vi "power_supply_FSM.vi"(0 "measurements q":refnum<queue>, 1 "commands q":refnum<queue>, 2 "GPIB":string, 3 "MAX_CURR":dbl, 4 "OUT_CURR":dbl, 5 "STEP":dbl=0.1, 7 "error in (no error)":errorcluster) -> ()   [LabVIEW 2019]
panel:
  out "state_and_args":string
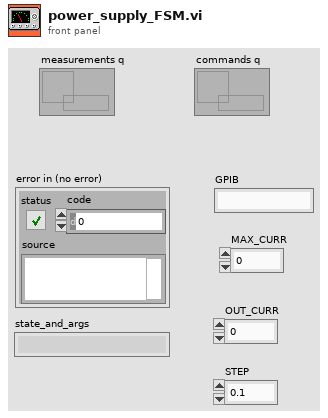
[diagram p1: front panel]
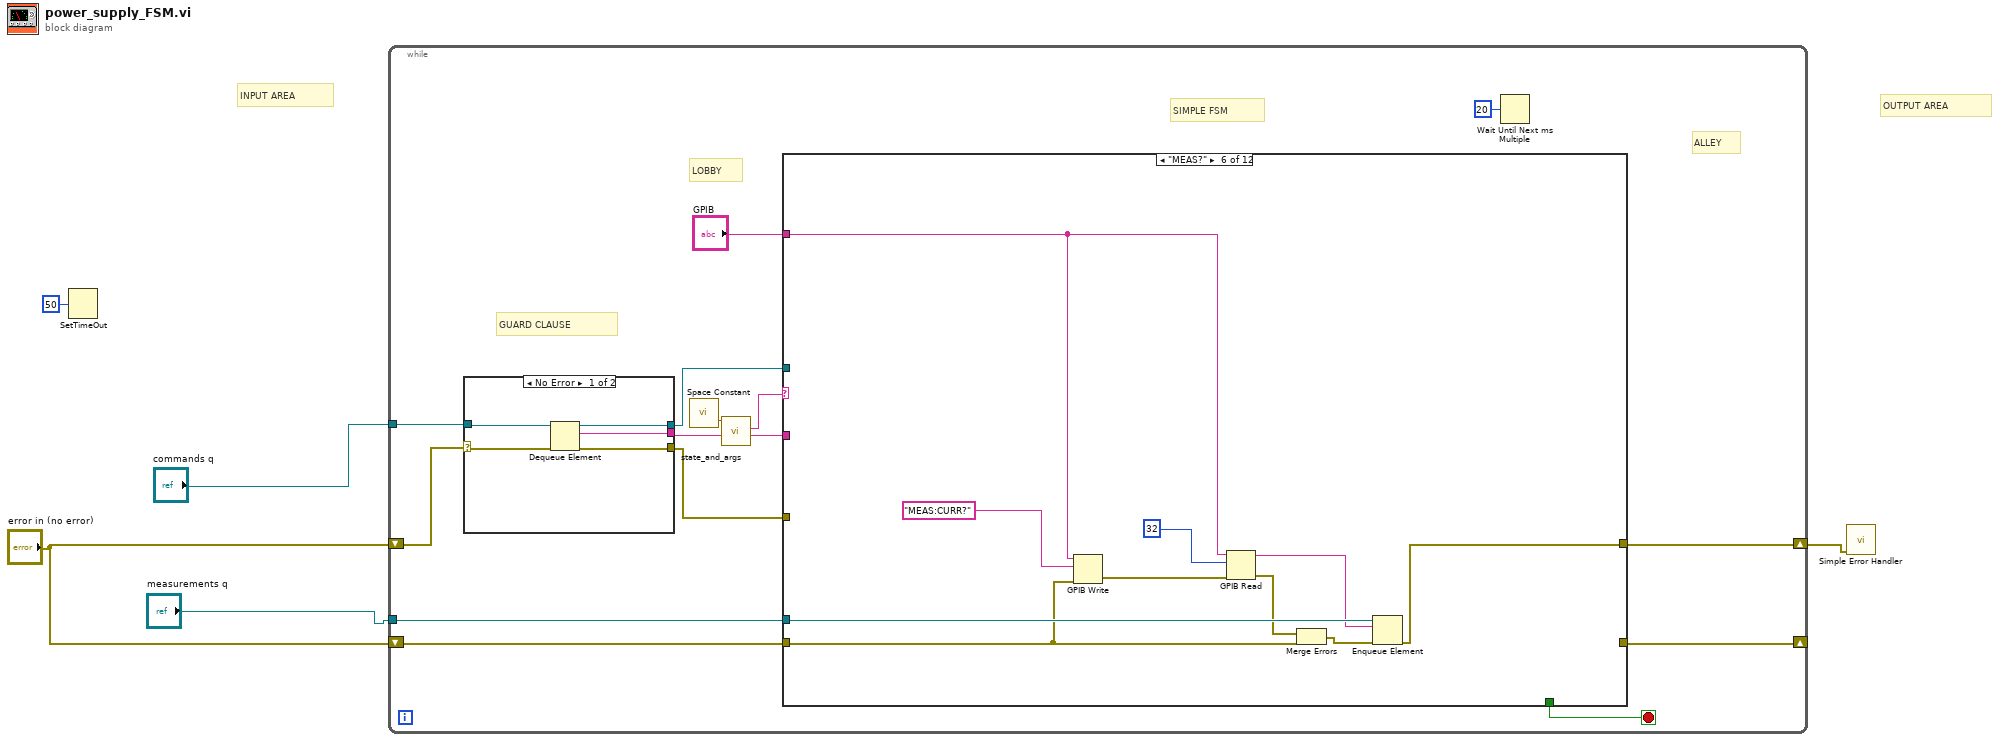
[diagram p0: block diagram]
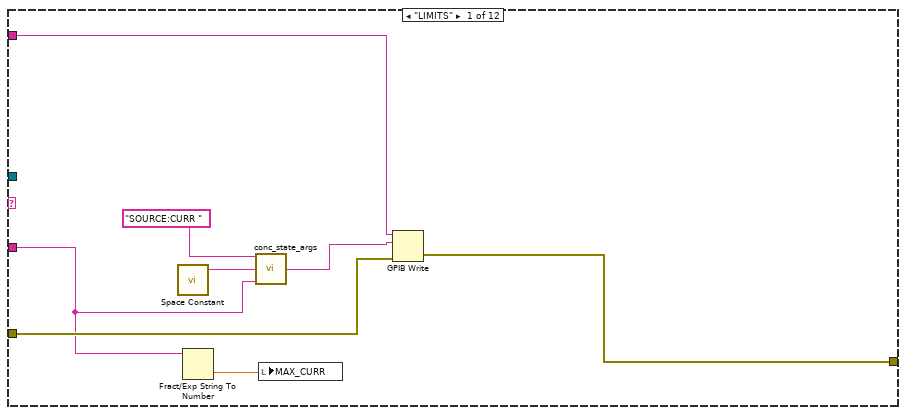
[diagram p2: hidden frame]
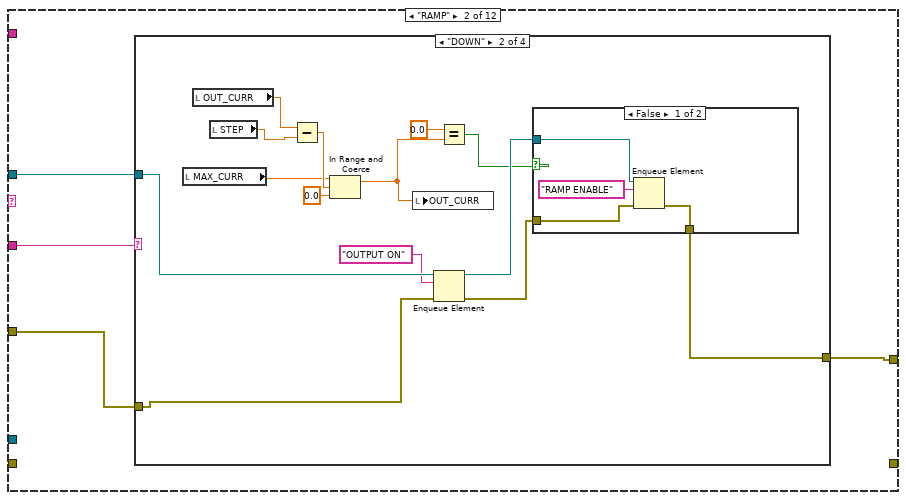
[diagram p3: hidden frame]
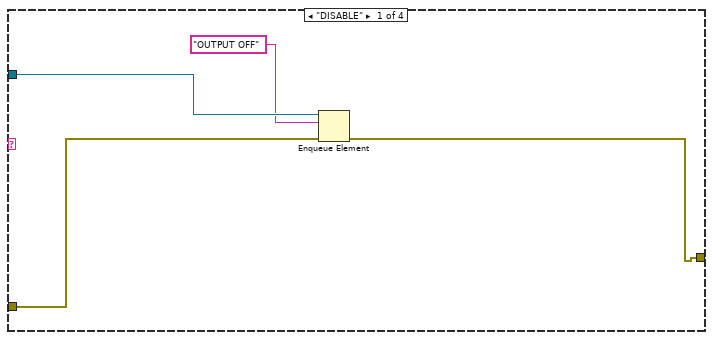
[diagram p4: hidden frame]
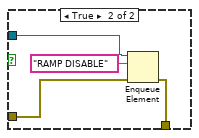
[diagram p5: hidden frame]
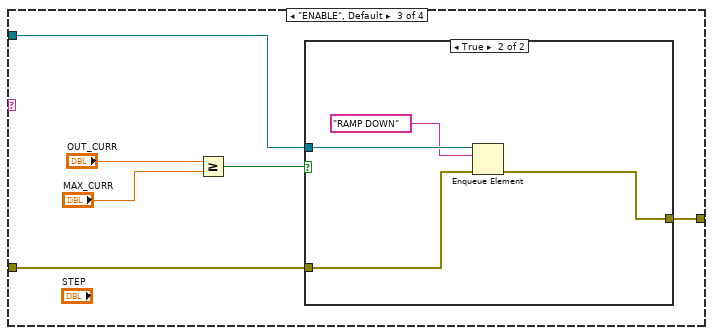
[diagram p6: hidden frame]
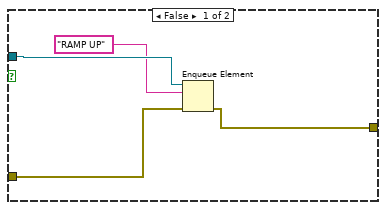
[diagram p7: hidden frame]
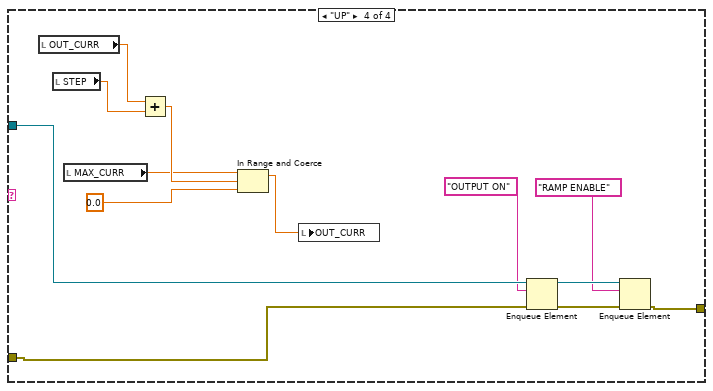
[diagram p8: hidden frame]
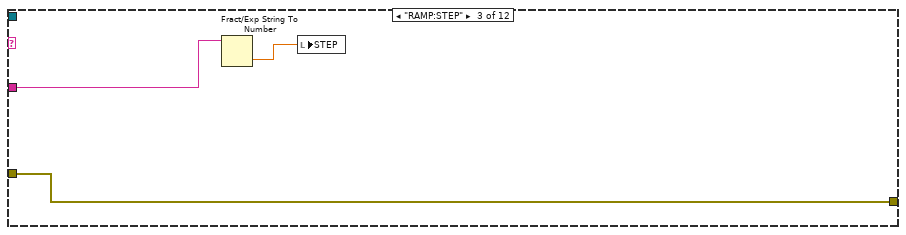
[diagram p9: hidden frame]
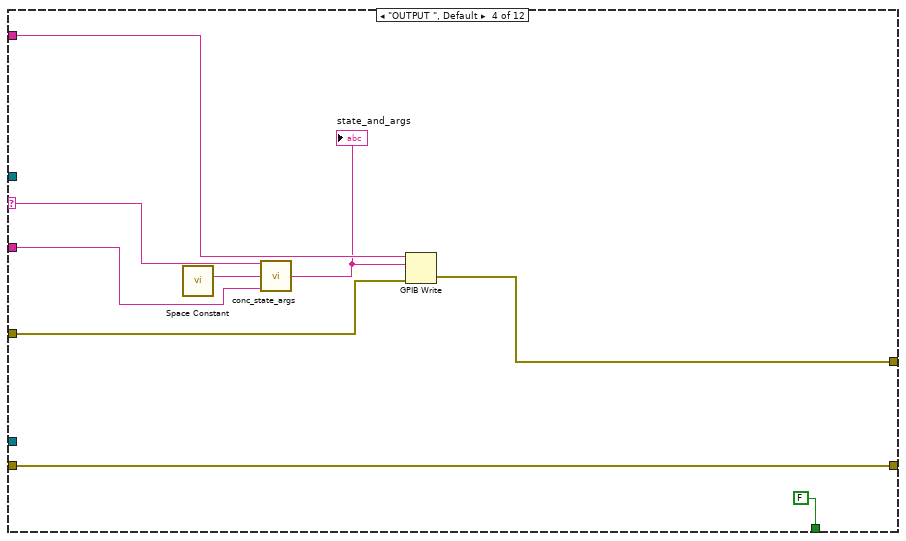
[diagram p10: hidden frame]
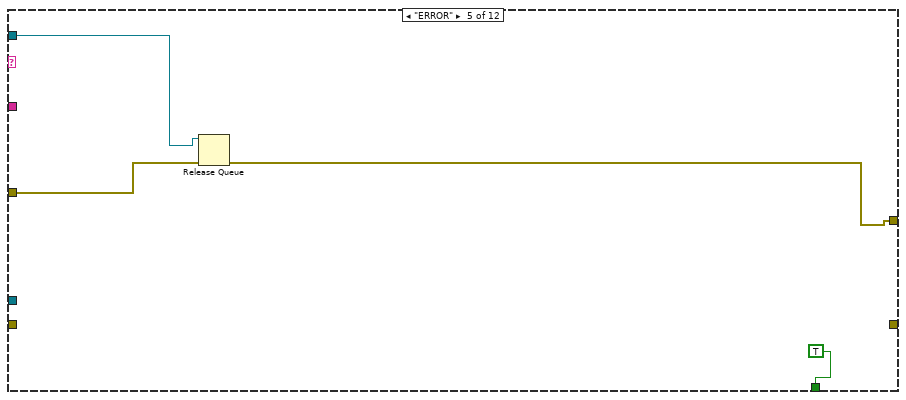
[diagram p11: hidden frame]
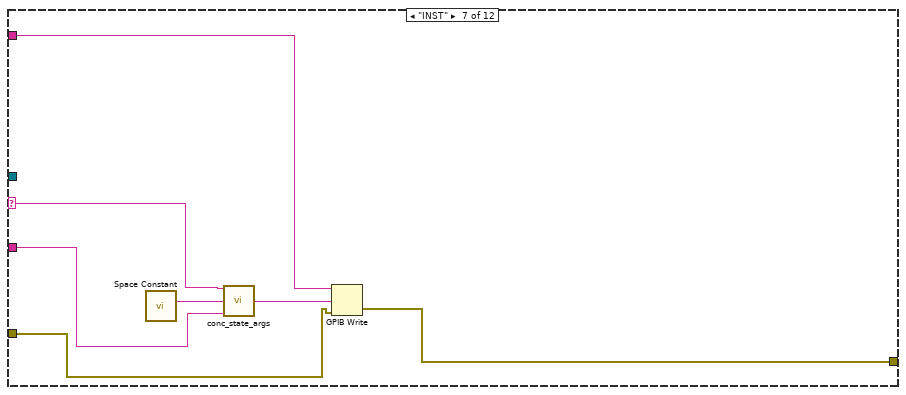
[diagram p12: hidden frame]
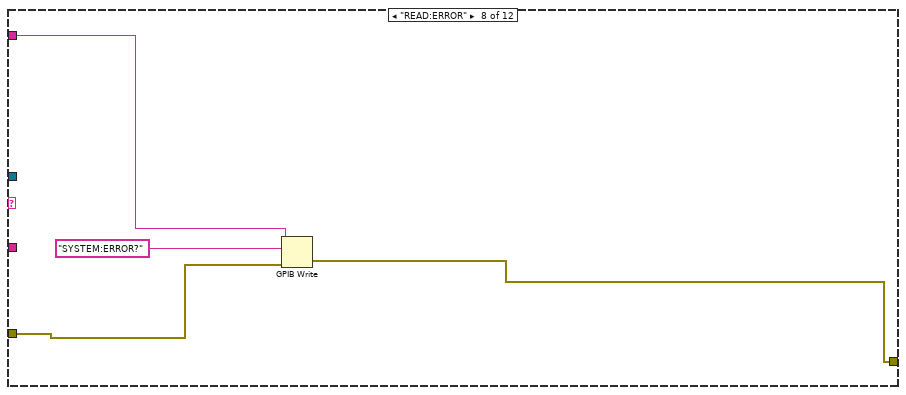
[diagram p13: hidden frame]
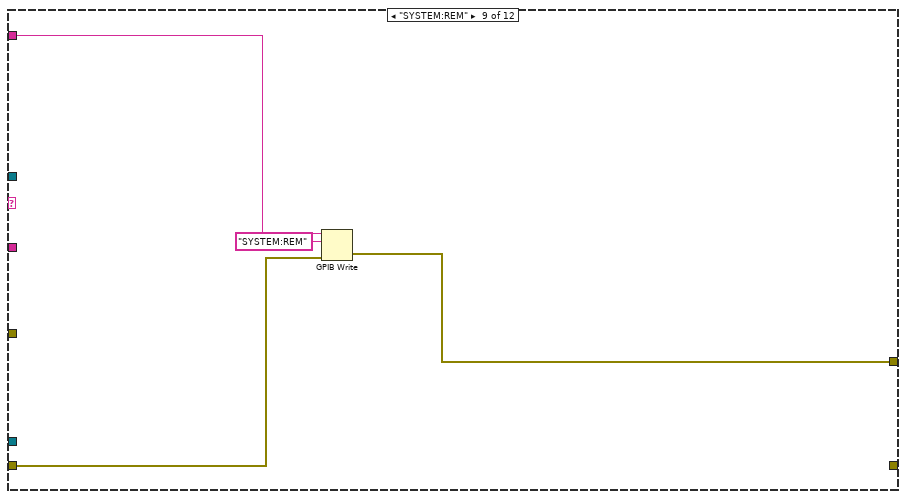
[diagram p14: hidden frame]
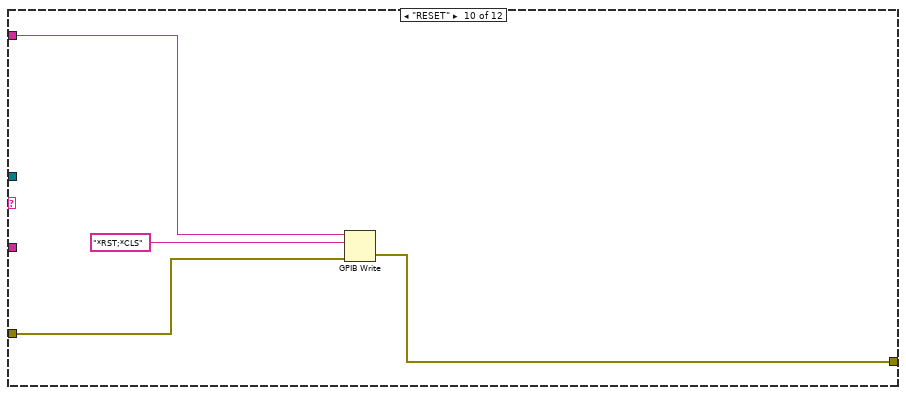
[diagram p15: hidden frame]
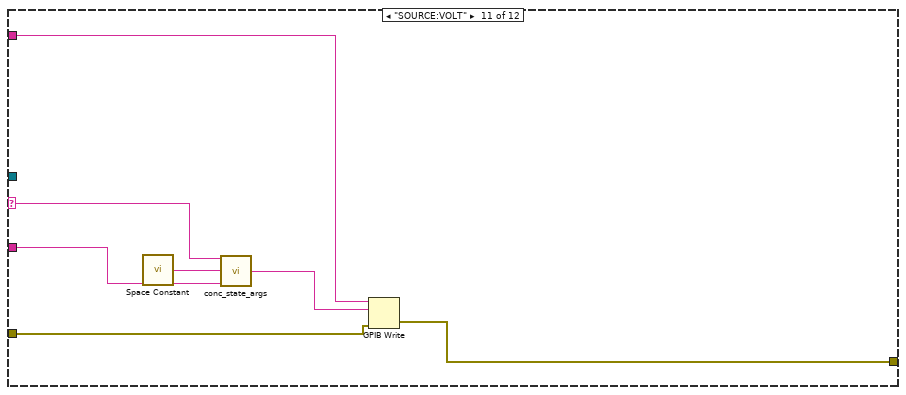
[diagram p16: hidden frame]
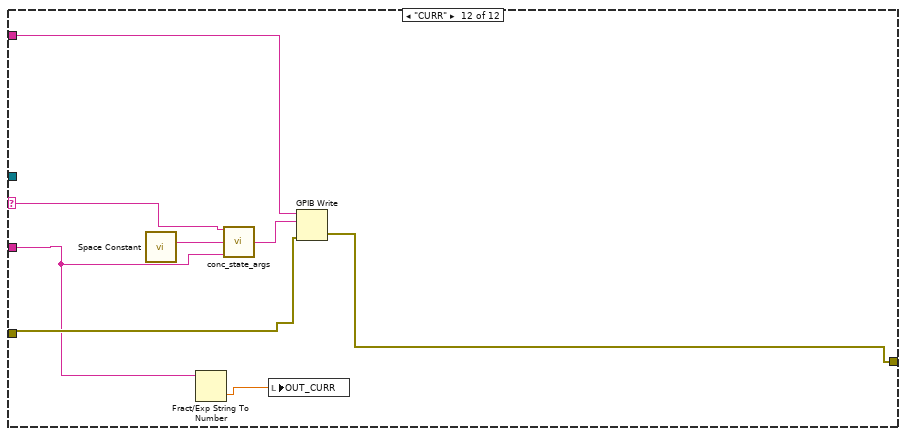
[diagram p17: hidden frame]
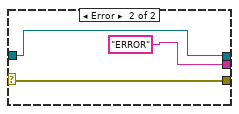
[diagram p18: hidden frame]
diagram:
  # "OUTPUT AREA"
  # "INPUT AREA"
  n1 = SetTimeOut(1:50 ("new timeout (10000)")) -> ()  [unwired: 1 out]
  n2 = while {
    tunnel: "commands q" -> [w19]
    shift-right: [w12] -> w4
    shift-left: "error in (no error)" -> [w20]
    shift-right: [w7] -> _
    shift-left: "error in (no error)" -> [w9]
    tunnel: "measurements q" -> [w8]
    stop <- w10 stop-if-true
    # "SIMPLE FSM"
    # "ALLEY"
    # "LOBBY"
    # "GUARD CLAUSE"
    n3 = case shown="No Error" w20 {
      selector: w20 -> [w149 w151]
      tunnel: w19 -> [w150 w152]
      tunnel: [w148 w152] -> w11
      tunnel: [w147 w151] -> w15
      tunnel: [w146 "ERROR"] -> w18
      frame No Error {
        n4 = Dequeue Element(queue=w150, error in (no error)=w149) -> (queue out=w148:refnum<queue>, element=w146:string, error out=w147:errorcluster)  [unwired: 1 in, 1 out]
      }
      frame Error {
      }
    }
    n5 = call <vilib>:"Space Constant.vi"() -> ("String"=w17:string)
    n6 = call "state_and_args.vi"("String"=w18, "DELIMITER (:)"=w17) -> ("Arguments"=w14:string, "State"=w16:string)  [unwired: 8 in]
    n7 = case shown="\"MEAS?\"" w16 {
      selector: w16 -> [_ _ _ w95 _ _ w115 _ _ _ w136 w143]
      tunnel: w15 -> [w25 w30 w86 w94 w100 _ w114 w120 _ w128 w132 w142]
      tunnel: w14 -> [w22 w32 w88 w97 _ _ w116 _ _ _ w137 w139]
      tunnel: "GPIB" -> [w26 _ _ w96 _ w110 w118 w122 w126 w130 w134 w145]
      tunnel: [w24 w29 w86 w93 w99 w106 w113 w119 w123 w127 w131 w141] -> w12
      tunnel: w11 -> [_ w31 _ _ w101 _ _ _ _ _ _ _]
      tunnel: [_ _ _ FALSE TRUE _ _ _ _ _ _ _] -> w10
      tunnel: w9 -> [_ _ _ w90 _ w105 _ _ w124 _ _ _]
      tunnel: w8 -> [_ _ _ _ _ w107 _ _ _ _ _ _]
      tunnel: [_ _ _ w90 _ _ _ _ _ _ _ _] -> w7
      frame "LIMITS" {
        n8 = call <vilib>:"Space Constant.vi"() -> ("String"=w28:string)
        n9 = Fract/Exp String To Number(string=w22) -> (number=w23:dbl)  [unwired: 3 in, 1 out]
        n10 = call "conc_state_args.vi"("State"="SOURCE:CURR ", "DELIMITER (:)"=w28, "Args"=w22) -> ("state_and_args"=w21:string)  [unwired: 12 in]
        n11 = local write "MAX_CURR"(w23) -> ()
        n12 = GPIB Write(0:w26, 1:w21, 3:w25) -> (6:w24:errorcluster)  [unwired: 2 in, 1 out]
      }
      frame "RAMP" {
        n13 = case shown="\"DOWN\"" w32 {
          tunnel: w31 -> [w36 w45 w60 w83]
          tunnel: w30 -> [w35 w44 w61 w82]
          tunnel: [w33 w37 w59 w77] -> w29
          frame "DISABLE" {
            n14 = Enqueue Element(queue=w36, element="OUTPUT OFF", error in (no error)=w35) -> (error out=w33:errorcluster)  [unwired: 1 in, 2 out]
          }
          frame "DOWN" {
            n15 = local read "MAX_CURR"() -> (w47:dbl)
            n16 = local read "OUT_CURR"() -> (w50:dbl)
            n17 = local read "STEP"() -> (w49:dbl)
            n18 = Subtract(x=w50, y=w49) -> (x-y=w48:dbl)
            n19 = In Range and Coerce(upper limit=w47, x=w48, lower limit=0.0) -> (coerced(x)=w42:dbl)  [unwired: 1 out]
            n20 = local write "OUT_CURR"(w42) -> ()
            n21 = Enqueue Element(queue=w45, element="OUTPUT ON", error in (no error)=w44) -> (queue out=w40:refnum<queue>, error out=w39:errorcluster)  [unwired: 1 in, 1 out]
            n22 = Equal?(x=0.0, y=w42) -> (x = y?=w38:bool)
            n23 = case shown="False" w38 {
              tunnel: w40 -> [w52 w58]
              tunnel: w39 -> [w53 w57]
              tunnel: [w54 w55] -> w37
              frame False {
                n24 = Enqueue Element(queue=w52, element="RAMP ENABLE", error in (no error)=w53) -> (error out=w54:errorcluster)  [unwired: 1 in, 2 out]
              }
              frame True {
                n25 = Enqueue Element(queue=w58, element="RAMP DISABLE", error in (no error)=w57) -> (error out=w55:errorcluster)  [unwired: 1 in, 2 out]
              }
            }
          }
          frame "ENABLE", Default {
            n26 = Greater Or Equal?(x="OUT_CURR", y="MAX_CURR") -> (x >= y?=w62:bool)
            n27 = case shown="True" w62 {
              tunnel: w61 -> [w67 w72]
              tunnel: w60 -> [w68 w71]
              tunnel: [w65 w69] -> w59
              frame False {
                n28 = Enqueue Element(queue=w68, element="RAMP UP", error in (no error)=w67) -> (error out=w65:errorcluster)  [unwired: 1 in, 2 out]
              }
              frame True {
                n29 = Enqueue Element(queue=w71, element="RAMP DOWN", error in (no error)=w72) -> (error out=w69:errorcluster)  [unwired: 1 in, 2 out]
              }
            }
          }
          frame "UP" {
            n30 = local read "OUT_CURR"() -> (w84:dbl)
            n31 = local read "STEP"() -> (w85:dbl)
            n32 = local read "MAX_CURR"() -> (w75:dbl)
            n33 = Add(x=w84, y=w85) -> (x+y=w76:dbl)
            n34 = In Range and Coerce(upper limit=w75, x=w76, lower limit=0.0) -> (coerced(x)=w73:dbl)  [unwired: 1 out]
            n35 = local write "OUT_CURR"(w73) -> ()
            n36 = Enqueue Element(queue=w83, element="OUTPUT ON", error in (no error)=w82) -> (queue out=w80:refnum<queue>, error out=w79:errorcluster)  [unwired: 1 in, 1 out]
            n37 = Enqueue Element(queue=w80, element="RAMP ENABLE", error in (no error)=w79) -> (error out=w77:errorcluster)  [unwired: 1 in, 2 out]
          }
        }
      }
      frame "RAMP:STEP" {
        n38 = Fract/Exp String To Number(string=w88) -> (number=w87:dbl)  [unwired: 3 in, 1 out]
        n39 = local write "STEP"(w87) -> ()
      }
      frame "OUTPUT ", Default {
        n40 = call <vilib>:"Space Constant.vi"() -> ("String"=w92:string)
        n41 = call "conc_state_args.vi"("State"=w95, "DELIMITER (:)"=w92, "Args"=w97) -> ("state_and_args"=w89:string)  [unwired: 12 in]
        "state_and_args" <- w89
        n42 = GPIB Write(0:w96, 1:w89, 3:w94) -> (6:w93:errorcluster)  [unwired: 2 in, 1 out]
      }
      frame "ERROR" {
        n43 = Release Queue(queue=w101, error in (no error)=w100) -> (error out=w99:errorcluster)  [unwired: 1 in, 2 out]
      }
      frame "MEAS?" {
        n44 = GPIB Write(0:w110, 1:"MEAS:CURR?", 3:w105) -> (6:w111:errorcluster)  [unwired: 2 in, 1 out]
        n45 = GPIB Read(0:w110, 1:32 ("byte count"), 3:w111) -> (5:w102:string, 7:w103:errorcluster)  [unwired: 2 in, 1 out]
        n46 = Merge Errors(w103, w105) -> (w108:errorcluster)
        n47 = Enqueue Element(queue=w107, element=w102, error in (no error)=w108) -> (error out=w106:errorcluster)  [unwired: 1 in, 2 out]
      }
      frame "INST" {
        n48 = call <vilib>:"Space Constant.vi"() -> ("String"=w117:string)
        n49 = call "conc_state_args.vi"("State"=w115, "DELIMITER (:)"=w117, "Args"=w116) -> ("state_and_args"=w112:string)  [unwired: 12 in]
        n50 = GPIB Write(0:w118, 1:w112, 3:w114) -> (6:w113:errorcluster)  [unwired: 2 in, 1 out]
      }
      frame "READ:ERROR" {
        n51 = GPIB Write(0:w122, 1:"SYSTEM:ERROR?" ("data"), 3:w120) -> (6:w119:errorcluster)  [unwired: 2 in, 1 out]
      }
      frame "SYSTEM:REM" {
        n52 = GPIB Write(0:w126, 1:"SYSTEM:REM" ("data"), 3:w124) -> (6:w123:errorcluster)  [unwired: 2 in, 1 out]
      }
      frame "RESET" {
        n53 = GPIB Write(0:w130, 1:"*RST;*CLS" ("data"), 3:w128) -> (6:w127:errorcluster)  [unwired: 2 in, 1 out]
      }
      frame "SOURCE:VOLT" {
        n54 = call <vilib>:"Space Constant.vi"() -> ("String"=w135:string)
        n55 = call "conc_state_args.vi"("State"=w136, "DELIMITER (:)"=w135, "Args"=w137) -> ("state_and_args"=w133:string)  [unwired: 12 in]
        n56 = GPIB Write(0:w134, 1:w133, 3:w132) -> (6:w131:errorcluster)  [unwired: 2 in, 1 out]
      }
      frame "CURR" {
        n57 = call <vilib>:"Space Constant.vi"() -> ("String"=w144:string)
        n58 = Fract/Exp String To Number(string=w139) -> (number=w140:dbl)  [unwired: 3 in, 1 out]
        n59 = call "conc_state_args.vi"("State"=w143, "DELIMITER (:)"=w144, "Args"=w139) -> ("state_and_args"=w138:string)  [unwired: 12 in]
        n60 = local write "OUT_CURR"(w140) -> ()
        n61 = GPIB Write(0:w145, 1:w138, 3:w142) -> (6:w141:errorcluster)  [unwired: 2 in, 1 out]
      }
    }
    n62 = Wait Until Next ms Multiple(millisecond multiple=u32 20) -> ()  [unwired: 1 out]
  }
  n63 = call <vilib>:"Simple Error Handler.vi"("error in (no error)"=w4) -> ()  [unwired: 4 in, 5 out]
